vi "Read RejectedCommand.vi"(8 "error in (no error)":errorcluster, 11 "ElectrometerController in":refnum<class "ElectrometerController.lvclass">) -> (0 "error out":errorcluster, 2 "RejectedCommand":refnum<user-event>, 3 "ElectrometerController out":refnum<class "ElectrometerController.lvclass">)   [LabVIEW 2016, in "ElectrometerController.lvclass"]
uses:
  ElectrometerController.lvclass
  ts_electrometeruserevents/PubSubDataEvent/PubSubDataEvent.lvclass
  ts_sallv_MtAtElectrometer/DataTypes/logevent_rejectedCommand.ctl
  ts_sallv_MtAtElectrometer/SALLV_MtAtElectrometer.lvlib
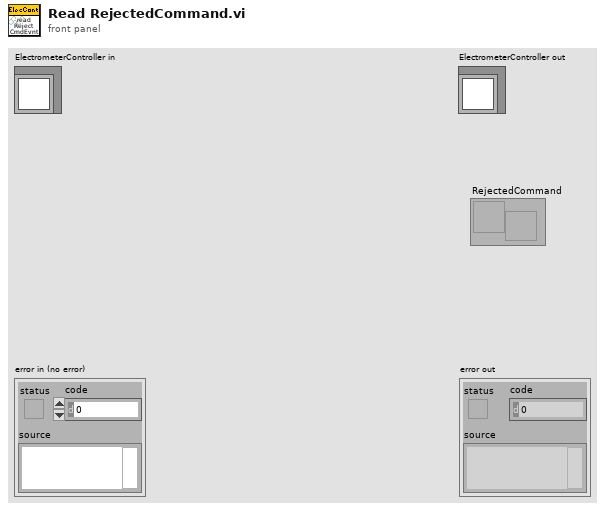
[diagram p1: front panel]
types:
  T1 = typedef "ElectrometerTypedefs.lvlib/PubDataEvents.ctl" = cluster{"ErrorCode":refnum<user-event>, "Heartbeat":refnum<user-event>, "LoopTime_ms":refnum<user-event>, "LoopTimeOutOfRange":refnum<user-event>, "RejectedCommand":refnum<user-event>, "SummaryState":refnum<user-event>, "Timestamp":refnum<user-event>, "AppliedSettingsMatchStart":refnum<user-event>, "InternalState":refnum<user-event>, "MeasureRange":refnum<user-event>, "DigitalFilterChange":refnum<user-event>, "MeasureType":refnum<user-event>, "Intensity":refnum<user-event>, "IntegrationTime":refnum<user-event>, "SettingsAppliedSerialConfiguration":refnum<user-event>, "SettingsAppliedReadingSettings":refnum<user-event>, "SettingVersions":refnum<user-event>, "LargeFileObjectAvailable":refnum<user-event>, "DetailedState":refnum<user-event>}
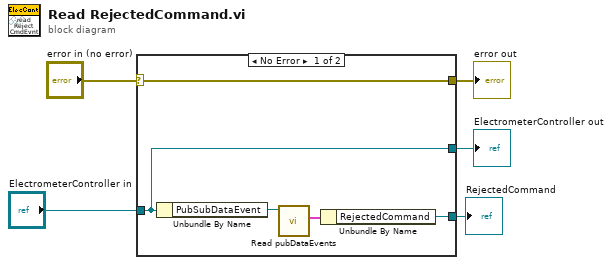
[diagram p0: block diagram]
diagram:
  n1 = case shown="No Error" "error in (no error)" {
    selector: "error in (no error)" -> [w10 w11]
    tunnel: [w10 w11] -> w4
    tunnel: [w9 w12] -> w2
    tunnel: "ElectrometerController in" -> [w9 w12]
    tunnel: [w6 _] -> w1
    frame No Error {
      n2 = Unbundle By Name(w9) -> ("PubSubDataEvent"=w8:refnum<class "PubSubDataEvent.lvclass">)
      n3 = call "Read pubDataEvents.vi"("PubSubDataEvent in"=w8) -> ("pubDataEvents"=w7:T1)  [unwired: 9 in, 1 out]
      n4 = Unbundle By Name(w7) -> ("RejectedCommand"=w6:refnum<user-event>)
    }
    frame Error {
    }
  }
  "error out" <- w4
  "ElectrometerController out" <- w2
  "RejectedCommand" <- w1
